vi "2-14.vi"() -> ()   [LabVIEW 2022 SP3]
panel:
  in  "温度下限值":dbl
  in  "温度上限值":dbl
  in  "停止":bool
  out "低温警示灯":bool
  out "高温警示灯":bool
  out "温度变化趋势图":T1(graph)
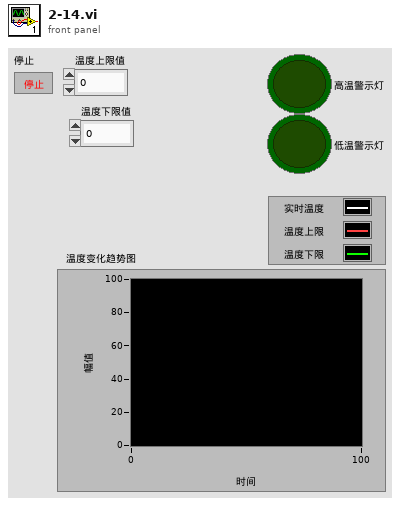
[diagram p1: front panel]
types:
  T1 = cluster{"Temperature":dbl, "温度上限值":dbl, "温度下限值":dbl}
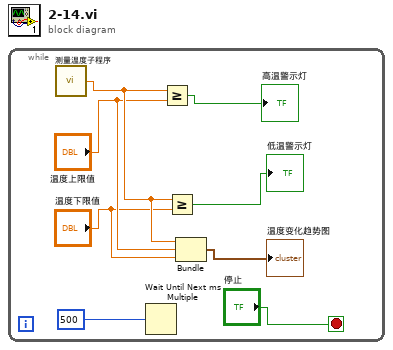
[diagram p0: block diagram]
diagram:
  n1 = while {
    stop <- "停止" stop-if-true
    n2 = call "测量温度子程序.vi"() -> ("Temperature"=w4:dbl)  [unwired: 1 in]
    n3 = Wait Until Next ms Multiple(millisecond multiple=500) -> ()  [unwired: 1 out]
    n4 = Greater Or Equal?(x=w4, y="温度上限值") -> (x >= y?=→"高温警示灯":bool)
    n5 = Greater Or Equal?(x=w4, y="温度下限值") -> (x >= y?=→"低温警示灯":bool)
    n6 = Bundle("Temperature"=w4, "温度上限值"="温度上限值", "温度下限值"="温度下限值") -> (→"温度变化趋势图":T1)  [unwired: 1 in]
  }
